vi "create IMAQ refrences.vi"(8 "error in (no error)":errorcluster, 11 "Cascade in":refnum<class "Cascade.lvclass">) -> (0 "error out":errorcluster, 3 "Cascade out":refnum<class "Cascade.lvclass">)   [LabVIEW 2012, in "Cascade.lvclass"]
uses:
  Cascade.lvclass
  Cascade.lvclass/Cascade.ctl
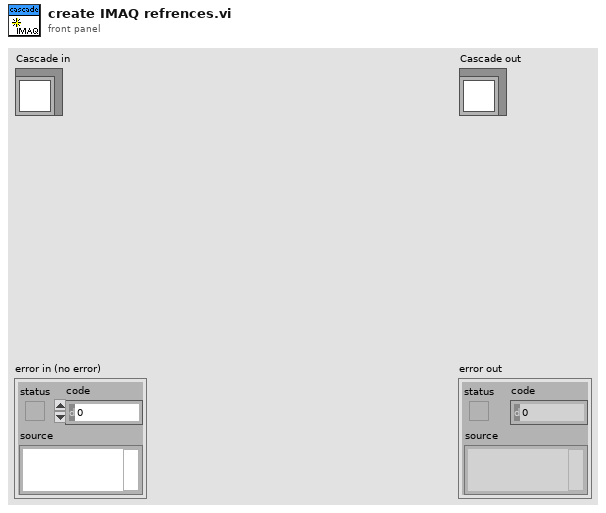
[diagram p1: front panel]
types:
  T1 = typedef "Image Type" = u32
  T2 = typedef "IMAQ Image.ctl" = refnum<image>
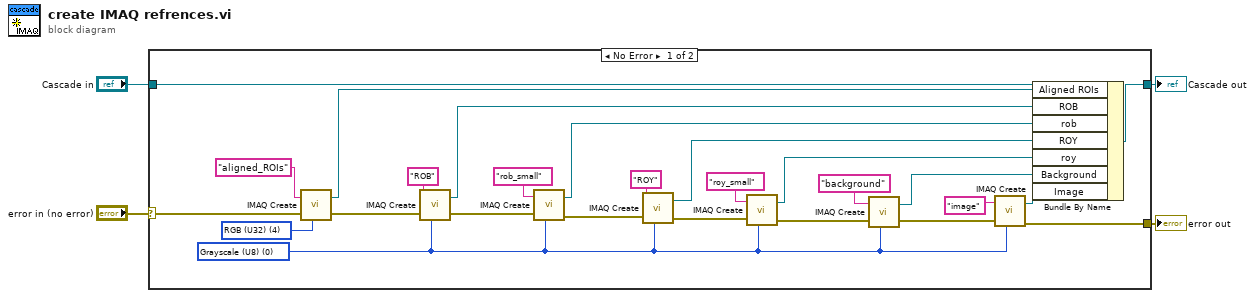
[diagram p0: block diagram]
diagram:
  n1 = case shown="No Error" "error in (no error)" {
    selector: "error in (no error)" -> [w9 w32]
    tunnel: [w26 w32] -> w3
    tunnel: [w24 w31] -> w1
    tunnel: "Cascade in" -> [w25 w31]
    frame No Error {
      w5 = T1 4 items=["Grayscale (U8)", "Grayscale (I16)", "Grayscale (SGL)", "Complex (CSG)", "RGB (U32)", "HSL (U32)", "RGB (U64)", "Grayscale (U16)"] ("Image Type")
      w14 = T1 0 items=["Grayscale (U8)", "Grayscale (I16)", "Grayscale (SGL)", "Complex (CSG)", "RGB (U32)", "HSL (U32)", "RGB (U64)", "Grayscale (U16)"] ("Image Type")
      n2 = call "IMAQ Create"("Image Name"="aligned_ROIs", "Image Type"=w5, "error in (no error)"=w9) -> ("New Image"=w6:T2, "error out"=w8:errorcluster)  [unwired: 2 in]
      n3 = call "IMAQ Create"("Image Name"="ROB", "Image Type"=w14, "error in (no error)"=w8) -> ("New Image"=w10:T2, "error out"=w15:errorcluster)  [unwired: 2 in]
      n4 = call "IMAQ Create"("Image Name"="rob_small", "Image Type"=w14, "error in (no error)"=w15) -> ("New Image"=w11:T2, "error out"=w16:errorcluster)  [unwired: 2 in]
      n5 = call "IMAQ Create"("Image Name"="ROY", "Image Type"=w14, "error in (no error)"=w16) -> ("New Image"=w12:T2, "error out"=w17:errorcluster)  [unwired: 2 in]
      n6 = call "IMAQ Create"("Image Name"="roy_small", "Image Type"=w14, "error in (no error)"=w17) -> ("New Image"=w13:T2, "error out"=w18:errorcluster)  [unwired: 2 in]
      n7 = call "IMAQ Create"("Image Name"="background", "Image Type"=w14, "error in (no error)"=w18) -> ("New Image"=w23:T2, "error out"=w27:errorcluster)  [unwired: 2 in]
      n8 = call "IMAQ Create"("Image Name"="image", "Image Type"=w14, "error in (no error)"=w27) -> ("New Image"=w30:T2, "error out"=w26:errorcluster)  [unwired: 2 in]
      n9 = Bundle By Name(cluster=w25, "Aligned ROIs"=w6, "ROB"=w10, "rob"=w11, "ROY"=w12, "roy"=w13, "Background"=w23, "Image"=w30) -> (w24:refnum<class "Cascade.lvclass">)
    }
    frame Error {
    }
  }
  "error out" <- w3
  "Cascade out" <- w1
